vi "NaN-Standard Deviation.vi"(4 "Array":dbl[](array[numeric])) -> (1 "NaN Std Dev":dbl, 2 "mean":dbl format="%0.2f")   [LabVIEW 2020]
uses:
  <vilib>/Analysis/NI_AALBase.lvlib
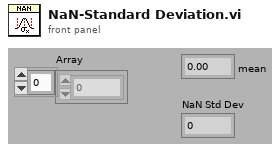
[diagram p1: front panel]
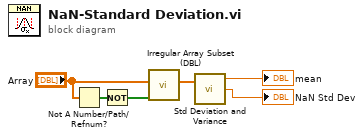
[diagram p0: block diagram]
diagram:
  n1 = Not A Number/Path/Refnum?(number/path/refnum="Array") -> (NaN/Path/Refnum?=w4:bool[])
  n2 = Not(x=w4) -> (.not. x?=w3:bool[])
  n3 = call "Irregular Array Subset (DBL).vi"("Mask"=w3, "Array"="Array") -> ("Array Subset"=w2:dbl[])  [unwired: 8 in, 1 out]
  n4 = call <vilib>:"Std Deviation and Variance.vi"("X"=w2) -> ("mean"=→"mean":dbl, "standard deviation"=→"NaN Std Dev":dbl)  [unwired: 1 in, 1 out]
